vi "Create.vi"(8 "error in (no error)":errorcluster, 11 "Thread in":refnum<class "Thread.lvclass">) -> (0 "error out":errorcluster, 3 "Thread out":refnum<class "Thread.lvclass">)   [LabVIEW 2017, in "DSF Core.lvlib" / "Thread.lvclass"]
uses:
  Thread.lvclass
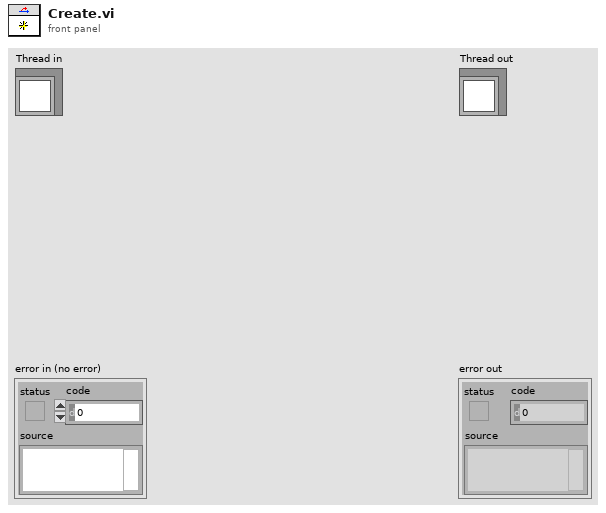
[diagram p1: front panel]
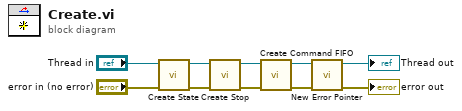
[diagram p0: block diagram]
diagram:
  n1 = call "Create State.vi"("error in (no error)"="error in (no error)", "Thread in"="Thread in") -> ("error out"=w8:errorcluster, "Thread out"=w7:refnum<class "Thread.lvclass">)  [unwired: 8 in]
  n2 = call "Create Stop.vi"("error in (no error)"=w8, "Thread in"=w7) -> ("error out"=w9:errorcluster, "Thread out"=w10:refnum<class "Thread.lvclass">)  [unwired: 8 in]
  n3 = call "Create Command FIFO.vi"("error in (no error)"=w9, "Thread in"=w10) -> ("error out"=w3:errorcluster, "Thread out"=w4:refnum<class "Thread.lvclass">)  [unwired: 8 in]
  n4 = call "New Error Pointer.vi"("error in (no error)"=w3, "Thread in"=w4) -> ("error out"=→"error out":errorcluster, "Thread out"=→"Thread out":refnum<class "Thread.lvclass">)  [unwired: 8 in]
